vi "Get Associated 5633 Resource Name from VST Resource Name.vi"(0 "VST Instrument Name":string, 5 "VST Channel":string, 11 "error in":errorcluster) -> (4 "5633 Resource Name":string, 6 "Found":bool, 15 "error out":errorcluster)   [LabVIEW 2023, in "RFCalAndFixtureCharact.Common.lvlib"]
uses:
  <vilib>/Utility/error.llb/Trim Whitespace One-Sided.vi
  <vilib>/Utility/error.llb/Error Cluster From Error Code.vi
  <vilib>/nisyscfg/Close (Resources).vi
  <vilib>/nisyscfg/Close (Filter).vi
  <vilib>/nisyscfg/Close (System).vi
  RFCalAndFixtureCharact.Common.lvlib
  <vilib>/nisyscfg/nisyscfg.lvlib
  <resource>/objmgr/niflexrioatomicsae.rc
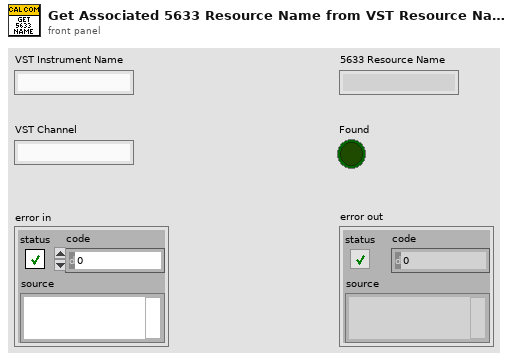
[diagram p1: front panel]
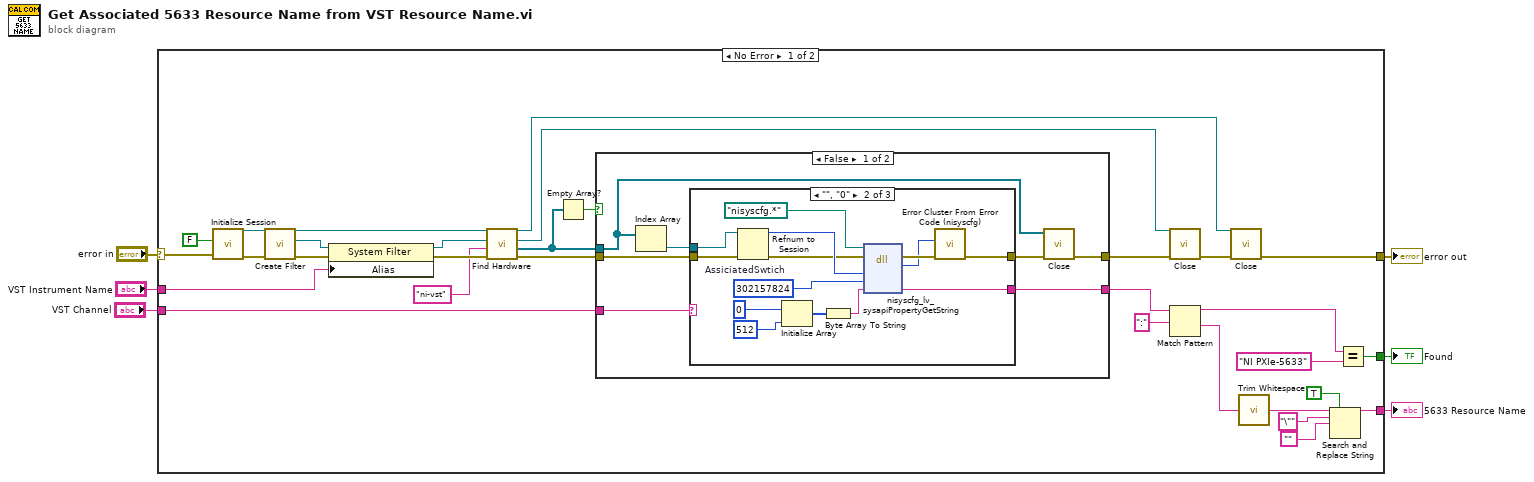
[diagram p0: block diagram]
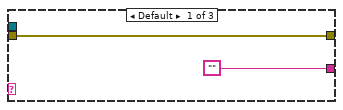
[diagram p2: hidden frame]
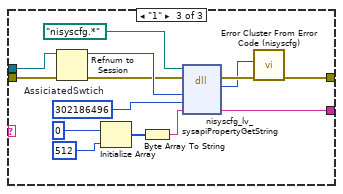
[diagram p3: hidden frame]
diagram:
  n1 = case shown="No Error" "error in" {
    selector: "error in" -> [w8 w76]
    tunnel: "VST Instrument Name" -> [w30 _]
    tunnel: [w26 w76] -> w5
    tunnel: [w18 _] -> w4
    tunnel: [w11 _] -> w3
    tunnel: "VST Channel" -> [w7 _]
    frame No Error {
      n2 = call <vilib>:"Initialize Session.vi"("error in (no error)"=w8, "Force Property Refresh (T)"=FALSE) -> ("error out"=w36:errorcluster, "Session out"=w35:refnum<k21>)  [unwired: 8 in]
      n3 = call <vilib>:"Create Filter.vi"("error in (no error)"=w36, "Session in"=w35) -> ("error out"=w37:errorcluster, "Filter out"=w10:refnum<k20>, "Session out"=w33:refnum<k21>)  [unwired: 7 in]
      n4 = property class="System Filter"(reference=w10, error in=w37, "Alias"=w30) -> (reference out=w9:refnum<k20>, error out=w34:errorcluster)
      n5 = call <vilib>:"Find Hardware.vi"("error in (no error)"=w34, "Experts"="ni-vst", "Filter in"=w9, "Session in"=w33) -> ("error out"=w32:errorcluster, "Resources out"=w17:refnum<k20>[], "Filter out"=w29:refnum<k20>, "Session out"=w31:refnum<k21>)  [unwired: 4 in]
      n6 = Empty Array?(array=w17) -> (empty?=w16:bool)
      n7 = case shown="False" w16 {
        tunnel: w32 -> [w39 w75]
        tunnel: w17 -> [w43 _]
        tunnel: [w42 w75] -> w28
        tunnel: [w41 _] -> w19
        tunnel: w7 -> [w40 _]
        frame False {
          n8 = Index Array(array=w43) -> (element=w38:refnum<k20>)  [unwired: 1 in]
          n9 = case shown="\"\", \"0\"" w40 {
            tunnel: w39 -> [w46 w56 w70]
            tunnel: w38 -> [_ w54 w68]
            tunnel: [w46 w55 w69] -> w44
            tunnel: ["" w48 w62] -> w41
            frame Default {
            }
            frame "", "0" {
              w52 = 302157824  # AssiciatedSwtich
              n10 = Refnum to Session(4:w56, 7:w54) -> (0:w59:errorcluster, 3:w60:u64)
              n11 = Initialize Array(u8 0, 512) -> (w50:u8[])
              n12 = Byte Array To String(unsigned byte array=w50) -> (string=w49:string)
              n13 = dll-call lib="nisyscfg.*" fn="nisyscfg_lv_sysapiPropertyGetString" ("CLN")(path in=path "nisyscfg.*", error in=w59, "object"=w60, "tag"=w52, "value"=w49) -> (error out=w58:errorcluster, "status"=w57:i32, "value"=w48:string)  [unwired: 3 in, 1 out]
              n14 = call <vilib>:"Error Cluster From Error Code (nisyscfg).vi"("error in (no error)"=w58, "Error Code (0)"=w57) -> ("error out"=w55:errorcluster)  [unwired: 9 in]
            }
            frame "1" {
              w66 = 302186496  # AssiciatedSwtich
              n15 = Refnum to Session(4:w70, 7:w68) -> (0:w73:errorcluster, 3:w74:u64)
              n16 = Initialize Array(u8 0, 512 ("dimension size")) -> (w64:u8[])
              n17 = Byte Array To String(unsigned byte array=w64) -> (string=w63:string)
              n18 = dll-call lib="nisyscfg.*" fn="nisyscfg_lv_sysapiPropertyGetString" ("CLN")(path in=path "nisyscfg.*", error in=w73, "object"=w74, "tag"=w66, "value"=w63) -> (error out=w72:errorcluster, "status"=w71:i32, "value"=w62:string)  [unwired: 3 in, 1 out]
              n19 = call <vilib>:"Error Cluster From Error Code (nisyscfg).vi"("error in (no error)"=w72, "Error Code (0)"=w71) -> ("error out"=w69:errorcluster)  [unwired: 9 in]
            }
          }
          n20 = call-poly <vilib>:"Close.vi"("error in (no error)"=w44, "Resources in"=w43) -> ("error out"=w42:errorcluster)  [unwired: 9 in]
        }
        frame True {
        }
      }
      n21 = call-poly <vilib>:"Close.vi"("error in (no error)"=w28, "Filter in"=w29) -> ("error out"=w27:errorcluster)  [unwired: 9 in]
      n22 = Match Pattern(string=w19, regular expression=":" ("search string/char (-)")) -> (before substring=w13:string, after substring=w20:string)  [unwired: 1 in, 2 out]
      n23 = call-poly <vilib>:"Close.vi"("error in (no error)"=w27, "Session in"=w31) -> ("error out"=w26:errorcluster)  [unwired: 9 in]
      n24 = call <vilib>:"Trim Whitespace.vi"("string"=w20) -> ("trimmed string"=w21:string)  [unwired: 1 in]
      n25 = Search and Replace String(replace all?=TRUE ("replace all? (F)"), input string=w21, search string="\"" ("search string/char (-)"), replace string="") -> (result string=w18:string)  [unwired: 4 in, 3 out]
      n26 = Equal?(x=w13, y="NI PXIe-5633") -> (x = y?=w11:bool)
    }
    frame Error {
    }
  }
  "error out" <- w5
  "5633 Resource Name" <- w4
  "Found" <- w3
